vi "Do Calculation.vi"(8 "error in (no error)":errorcluster, 10 "Array":T1[](array[typedef]) {"Zoom Parameters"."fwidth:" format="%#_6p"; "Zoom Parameters"."f0:" format="%#_6p"}, 11 "GPU FFT Calculator in":refnum<class "GPU FFT Calculator.lvclass">) -> (0 "error out":errorcluster, 3 "GPU FFT Calculator out":refnum<class "GPU FFT Calculator.lvclass">)   [LabVIEW 2020, in "GPU FFT Calculator.lvlib" / "GPU FFT Calculator.lvclass"]
uses:
  GPU FFT Calculator.lvclass
  C:/Users/natan/Documents/G2CPU-Performance-Demo/Calculation Worker/Calculation Worker/Calculation Worker.lvclass
  GPU Calculation Message.ctl
  <vilib>/Natan Biesmans/G2CPU GPU and CPU HPC Toolkit/G2CPU Libraries/Async IO/DMA Manager/DMA Manager.lvclass
  <vilib>/Natan Biesmans/G2CPU GPU and CPU HPC Toolkit/G2CPU Libraries/Arrays/1DArray/s16/1D Array s16.lvclass
  <vilib>/Natan Biesmans/G2CPU GPU and CPU HPC Toolkit/G2CPU Libraries/Arrays/1DArray/f32/1D Array f32.lvclass
  chart zoom.ctl
  GPU Metrics.ctl
  GPU FFT Calculator.lvclass/GPU FFT Calculator.ctl
  QMH Message.ctl
  Simple UI/Simple UI/Simple UI.lvclass
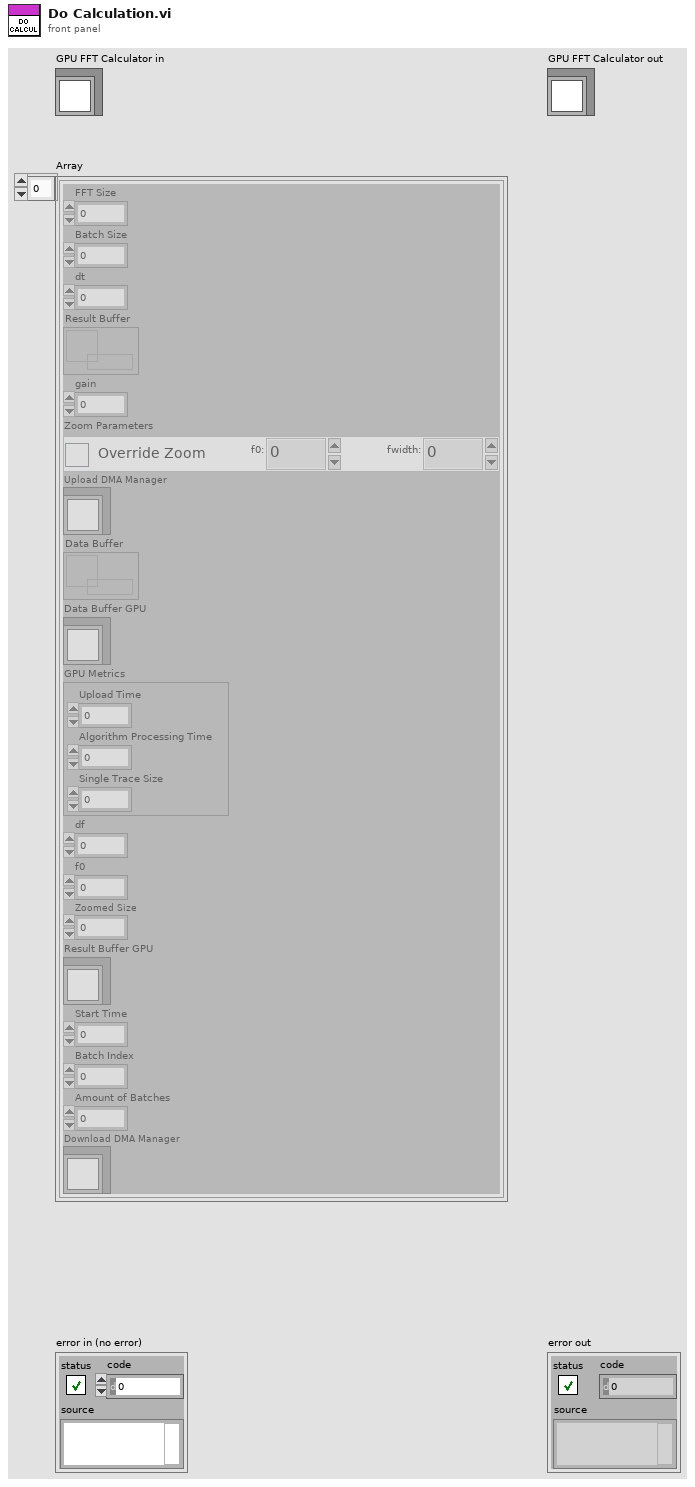
[diagram p1: front panel]
types:
  T1 = typedef "GPU FFT Calculator.lvlib/GPU FFT Calculator.lvclass/GPU Calculation Message.ctl" = cluster{"FFT Size":u64, "Batch Size":u64, "dt":dbl, "Result Buffer":refnum<data-value>, "gain":dbl, "Zoom Parameters":T2, "Upload DMA Manager":refnum<class "DMA Manager.lvclass">, "Data Buffer":refnum<data-value>, "Data Buffer GPU":refnum<class "1D Array s16.lvclass">, "GPU Metrics":T3, "df":dbl, "f0":dbl, "Zoomed Size":u64, "Result Buffer GPU":refnum<class "1D Array f32.lvclass">, "Start Time":dbl, "Batch Index":i32, "Amount of Batches":i32, "Download DMA Manager":refnum<class "DMA Manager.lvclass">}
  T2 = typedef "Simple UI.lvlib/Simple UI.lvclass/chart zoom.ctl" = cluster{"Override":bool, "f0: ":dbl, "fwidth: ":dbl}
  T3 = typedef "GPU FFT Calculator.lvlib/GPU FFT Calculator.lvclass/GPU Metrics.ctl" = cluster{"Upload Time":dbl, "Algorithm Processing Time":dbl, "Single Trace Size":u64}
  T4 = typedef "GPU FFT Calculator.lvlib/GPU FFT Calculator.lvclass/QMH Message.ctl" = cluster{"Command":string, "Data":variant}
  T5 = cluster{"Override":bool, "f0: ":bool, "fwidth: ":bool}
  T6 = typedef "Data Source.lvlib/Data Source.lvclass/Data Source Buffer.ctl" = refnum<data-value>
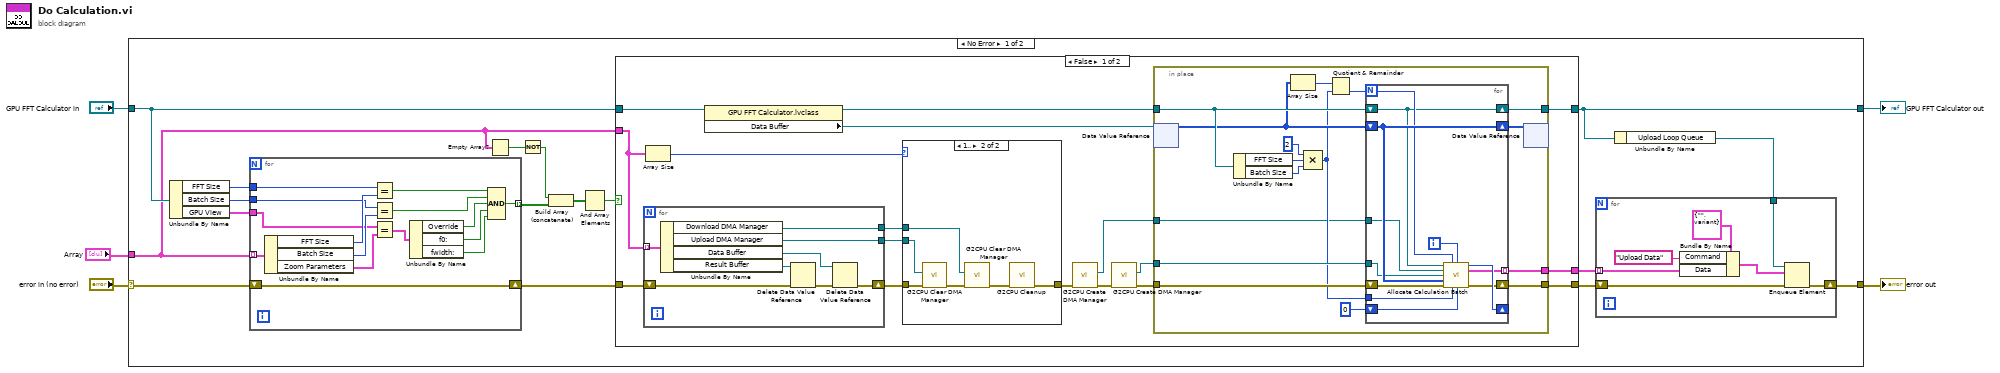
[diagram p0: block diagram]
diagram:
  n1 = case shown="No Error" "error in (no error)" {
    selector: "error in (no error)" -> [w18 w109]
    tunnel: [w22 w109] -> w4
    tunnel: [w21 w108] -> w2
    tunnel: "GPU FFT Calculator in" -> [w20 w108]
    tunnel: "Array" -> [w9 _]
    frame No Error {
      n2 = Unbundle By Name(w20) -> ("FFT Size"=w17:u64, "Batch Size"=w16:u64, "GPU View"=w15:T2)
      n3 = for {
        tunnel: w9 -> [w100] mode=indexing
        shift-right: [w93] -> w12
        shift-left: w18 -> [w93]
        tunnel: w17 -> [w99]
        tunnel: w16 -> [w97]
        tunnel: w15 -> [w94]
        tunnel: [w86] -> w14 mode=indexing
        n4 = Unbundle By Name(w100) -> ("FFT Size"=w98:u64, "Batch Size"=w96:u64, "Zoom Parameters"=w95:T2)
        n5 = Equal?(x=w99, y=w98) -> (x = y?=w91:bool)
        n6 = Equal?(x=w97, y=w96) -> (x = y?=w92:bool)
        n7 = Equal?(x=w94, y=w95) -> (x = y?=w90:T5)
        n8 = Unbundle By Name(w90) -> ("Override"=w87:bool, "f0:"=w88:bool, "fwidth:"=w89:bool)
        n9 = Compound Arithmetic op=AND(w91, w92, w87, w88, w89) -> (w86:bool)
      }
      n10 = Empty Array?(array=w9) -> (empty?=w8:bool)
      n11 = Not(x=w8) -> (.not. x?=w6:bool)
      n12 = Build Array (concatenate)(w6, w14) -> (w7:bool[])
      n13 = And Array Elements(Boolean array=w7) -> (logical AND=w13:bool)
      n14 = case shown="False" w13 {
        tunnel: [w31 w84] -> w21
        tunnel: w20 -> [w29 w84]
        tunnel: w12 -> [w39 w85]
        tunnel: w9 -> [w37 w83]
        tunnel: [w27 w85] -> w11
        tunnel: [w28 w83] -> w10
        frame False {
          n15 = for {
            tunnel: w37 -> [w82] mode=indexing
            tunnel: [w81] -> w35
            shift-right: [w76] -> w36
            shift-left: w39 -> [w78]
            tunnel: [w75] -> w26
            n16 = Unbundle By Name(w82) -> ("Download DMA Manager"=w75:refnum<class "DMA Manager.lvclass">, "Upload DMA Manager"=w81:refnum<class "DMA Manager.lvclass">, "Data Buffer"=w79:refnum<data-value>, "Result Buffer"=w80:refnum<data-value>)
            n17 = Delete Data Value Reference(data value reference=w80, error in=w78) -> (error out=w77:errorcluster)  [unwired: 1 out]
            n18 = Delete Data Value Reference(data value reference=w79, error in=w77) -> (error out=w76:errorcluster)  [unwired: 1 out]
          }
          n19 = Array Size(array=w37) -> (size(s)=w38:i32)
          n20 = property class="GPU FFT Calculator.lvclass"(reference=w29) -> (reference out=w30:refnum<class "GPU FFT Calculator.lvclass">, "Data Buffer"=w34:T6)  [unwired: 1 in, 1 out]
          n21 = case shown="1.." w38 {
            tunnel: w36 -> [w68 w73]
            tunnel: w35 -> [_ w74]
            tunnel: [w68 w69] -> w25
            tunnel: w26 -> [_ w70]
            frame Default {
            }
            frame 1.. {
              n22 = call <vilib>:"G2CPU Clear DMA Manager.vi"("error in (no error)"=w73, "DMA Manager"=w74) -> ("error out"=w72:errorcluster)  [unwired: 9 in]
              n23 = call <vilib>:"G2CPU Clear DMA Manager.vi"("error in (no error)"=w72, "DMA Manager"=w70) -> ("error out"=w71:errorcluster)  [unwired: 9 in]
              n24 = call <vilib>:"G2CPU Cleanup.vi"("error in (no error)"=w71) -> ("error out"=w69:errorcluster)  [unwired: 10 in]
            }
          }
          n25 = call <vilib>:"G2CPU Create DMA Manager.vi"("error in (no error)"=w25) -> ("error out"=w24:errorcluster, "DMA Manager"=w23:refnum<class "DMA Manager.lvclass">)  [unwired: 9 in]
          n26 = call <vilib>:"G2CPU Create DMA Manager.vi"("error in (no error)"=w24) -> ("error out"=w33:errorcluster, "DMA Manager"=w32:refnum<class "DMA Manager.lvclass">)  [unwired: 9 in]
          n27 = in-place {
            in-place-border: w33 -> [w55]
            in-place-border: w32 -> [w54]
            in-place-border: [w52] -> w31
            in-place-border: w30 -> [w51]
            in-place-border: [w42] -> w28
            in-place-border: [w41] -> w27
            in-place-border: w23 -> [w40]
            n28 = in-place-dvr #1(w34) -> (w46:i16[])  [unwired: 1 out]
            n29 = Unbundle By Name(w51) -> ("FFT Size"=w49:u64, "Batch Size"=w48:u64)
            n30 = Array Size(array=w46) -> (size(s)=w45:i32)
            n31 = Compound Arithmetic op=MULTIPLY(u64 2 ("value"), w49, w48) -> (w44:u64)
            n32 = Quotient & Remainder(x=w45, y=w44) -> (floor(x/y)=w43:u64)  [unwired: 1 out]
            n33 = for {
              N: w43 -> [w61]
              tunnel: w54 -> [w60]
              shift-right: [w65] -> w53
              shift-left: w46 -> [w65]
              shift-right: [w59] -> w52
              shift-left: w51 -> [w59]
              shift-right: [w66] -> _
              shift-left: u64 0 ("value") -> [w67]
              tunnel: w44 -> [w63]
              tunnel: [w64] -> w42 mode=indexing
              shift-right: [w58] -> w41
              shift-left: w55 -> [w57]
              tunnel: w40 -> [w56]
              i -> [w62]
              n34 = call "Allocate Calculation Batch.vi"("GPU FFT Calculator in"=w59, "Amount of Batches"=w61, "Batch Index"=w62, "Download DMA Manager"=w56, "Upload DMA Manager"=w60, "Dataset"=w65, "error in (no error)"=w57, "Frame Size"=w63, "Data Offset In"=w67) -> ("Data Offset Out"=w66:u64, "Calculation Batch"=w64:T1, "error out"=w58:errorcluster)  [unwired: 4 in]
            }
            n35 = in-place-dvr #1(w53) -> ()  [unwired: 2 out]
          }
        }
        frame True {
        }
      }
      n36 = Unbundle By Name(w21) -> ("Upload Loop Queue"=w19:refnum<queue>)
      n37 = for {
        tunnel: w19 -> [w106]
        shift-right: [w107] -> w22
        shift-left: w11 -> [w102]
        tunnel: w10 -> [w101] mode=indexing
        n38 = Bundle By Name(cluster=T4 {"Command"="", "Data"=variant} ("Cluster"), "Command"="Upload Data", "Data"=w101) -> (w104:T4)
        n39 = Enqueue Element(queue=w106, element=w104, error in (no error)=w102) -> (error out=w107:errorcluster)  [unwired: 1 in, 2 out]
      }
    }
    frame Error {
    }
  }
  "error out" <- w4
  "GPU FFT Calculator out" <- w2
